vi "Normalize Decay v2.vi"(8 "Error In":errorcluster, 9 "Max = 1 (F)/Integral = 1 (T)":bool, 11 "Decay":cluster{"t Array":dbl[], "Y Array":dbl[]}) -> (0 "Error Out":errorcluster, 1 "Step":dbl, 2 "Normalization Factor":dbl, 3 "Normalized Decay":cluster{"t Array":dbl[], "Y Array":dbl[]}, 4 "Is Valid Plot?":bool)   [LabVIEW 2021, in "Fits.lvlib"]
doc: "Normalizes the incoming plot such that the integral equals 1.\n\n* <B>IRF = False</B>: The Y Array is divided by the sum of all Y values (<B>Normalization Factor</B>) multiplied by the most likely abscissa step (<B>Step</B>, maximum interval between successive abscissa).\n\n* <B>IRF = True</B>: The Y Array is divided by the sum of all Y values (<B>Normalization Factor</B>)."
uses:
  Fits.lvlib
  c65b08c5-93fc-4e90-ad2d-ad135c1fbea9.vi
  Graphs/XY Graph/XY Graph Add-Ons.lvlib
  daa3c5e8-17f1-472d-9035-27f7e7097246.vi
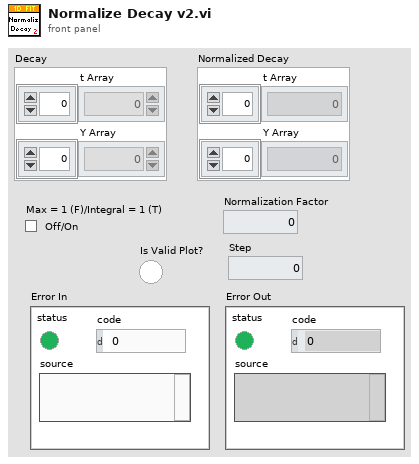
[diagram p1: front panel]
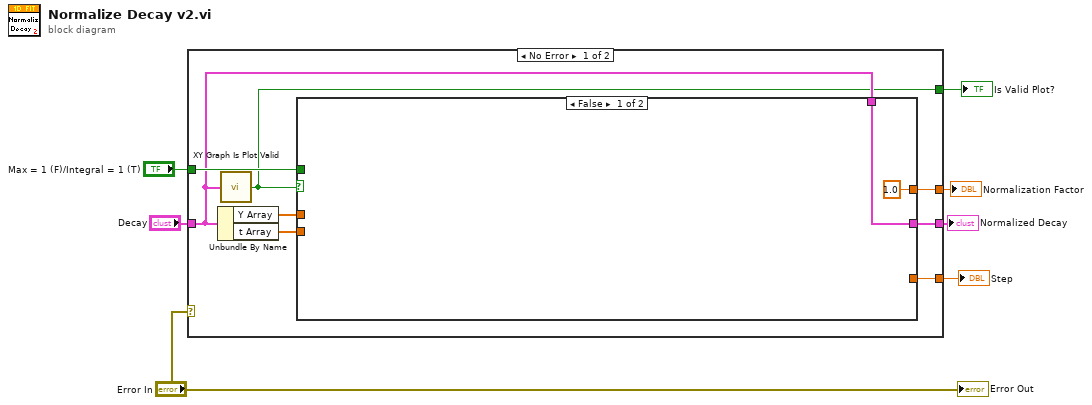
[diagram p0: block diagram]
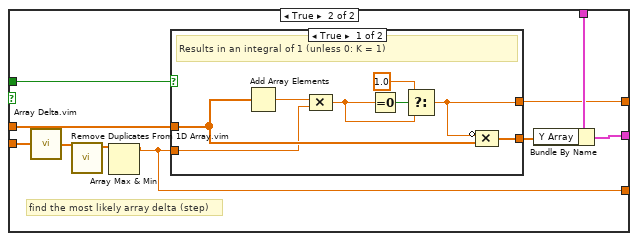
[diagram p2: hidden frame]
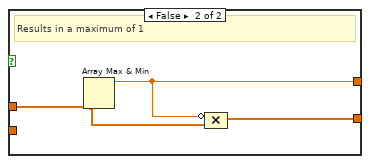
[diagram p3: hidden frame]
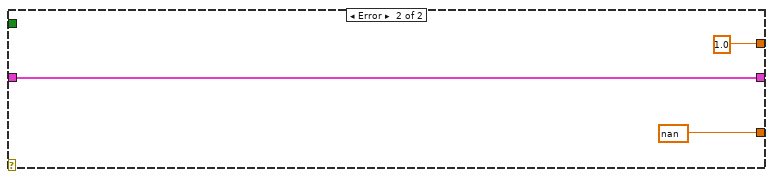
[diagram p4: hidden frame]
diagram:
  n1 = case shown="No Error" "Error In" {
    tunnel: "Decay" -> [w9 w41]
    tunnel: [w15 w41] -> w6
    tunnel: [w14 1.0 ("t")] -> w5
    tunnel: [w13 nan] -> w4
    tunnel: "Max = 1 (F)/Integral = 1 (T)" -> [w10 _]
    tunnel: [w8 _] -> w1
    frame No Error {
      n2 = Unbundle By Name(w9) -> ("Y Array"=w12:dbl[], "t Array"=w11:dbl[])
      n3 = call "XY Graph Is Plot Valid.vi"("Plot"=w9) -> ("Is Valid Plot?"=w8:bool)  [unwired: 8 in]
      n4 = case shown="False" w8 {
        tunnel: w9 -> [w16 w27]
        tunnel: [w16 w26] -> w15
        tunnel: w11 -> [_ w25]
        tunnel: w12 -> [_ w23]
        tunnel: [1.0 ("t") w22] -> w14
        tunnel: [_ w19] -> w13
        tunnel: w10 -> [_ w18]
        frame False {
        }
        frame True {
          # "find the most likely array delta (step)"
          n5 = call "Array Delta.vim"("A[i]"=w25) -> ("A[i+1]-A[i]"=w20:dbl[])  [unwired: 8 in]
          n6 = call "Remove Duplicates From 1D Array.vim"("array"=w20) -> ("array with duplicates removed"=w21:dbl[])  [unwired: 10 in]
          n7 = Array Max & Min(array=w21) -> (max value=w19:dbl)  [unwired: 3 out]
          n8 = case shown="True" w18 {
            tunnel: [w35 w38] -> w24
            tunnel: w23 -> [w34 w37]
            tunnel: [w28 w36] -> w22
            tunnel: w19 -> [w31 _]
            frame True {
              # "Results in an integral of 1 (unless 0: K = 1)"
              n9 = Add Array Elements(numeric array=w34) -> (sum=w30:dbl)
              n10 = Compound Arithmetic op=MULTIPLY(w30, w31) -> (w29:dbl)
              n11 = Equal To 0?(x=w29) -> (x = 0?=w33:bool)
              n12 = Select(t=1.0, s=w33, f=w29) -> (s? t:f=w28:dbl)
              n13 = Compound Arithmetic op=MULTIPLY(invert w28, w34) -> (w35:dbl[])
            }
            frame False {
              # "find the most likely array delta (step)"
              # "Results in a maximum of 1"
              n14 = Array Max & Min(array=w37) -> (max value=w36:dbl)  [unwired: 3 out]
              n15 = Compound Arithmetic op=MULTIPLY(invert w36, w37) -> (w38:dbl[])
            }
          }
          n16 = Bundle By Name(cluster=w27, "Y Array"=w24) -> (w26:cluster{"t Array":dbl[], "Y Array":dbl[]})
        }
      }
    }
    frame Error {
    }
  }
  "Normalized Decay" <- w6
  "Normalization Factor" <- w5
  "Step" <- w4
  "Is Valid Plot?" <- w1
  "Error Out" <- "Error In"
